vi "Get Enum Text.vi"(8 "error in (no error)":errorcluster, 11 "Enum":T1) -> (0 "error out":errorcluster, 3 "Enum Text":string)   [LabVIEW 2026]
uses:
  controls/UI/Measurement Role.ctl
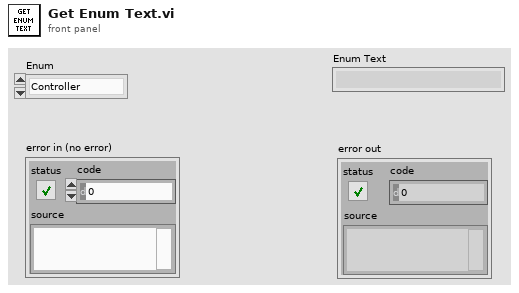
[diagram p1: front panel]
types:
  T1 = typedef "Measurement Role.ctl" = enum16{"Controller", "Reference", "UUT", "Disable"}
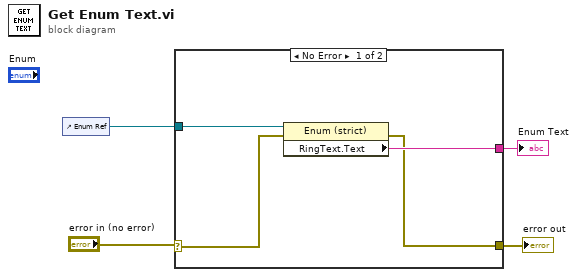
[diagram p0: block diagram]
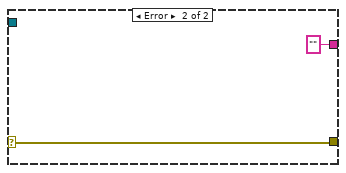
[diagram p2: hidden frame]
diagram:
  n1 = control-ref of="Enum Ref"() -> (w4:refnum<vi>)
  n2 = case shown="No Error" "error in (no error)" {
    selector: "error in (no error)" -> [w6 w10]
    tunnel: w4 -> [w8 _]
    tunnel: [w7 "" ("RingText.Text")] -> w3
    tunnel: [w5 w10] -> w1
    frame No Error {
      n3 = property class="Enum (strict)"(reference=w8, error in=w6) -> (error out=w5:errorcluster, "RingText.Text"=w7:string)  [unwired: 1 out]
    }
    frame Error {
    }
  }
  "Enum Text" <- w3
  "error out" <- w1
